vi "Logger.vi"() -> ()   [LabVIEW 2016]
uses:
  tools/CitTemplate/citTemplate.errData.ctl
  Logger.Action.ctl
  Sequence/Sequence.State.ctl
  Sequence/Sequence.Step.Status.ctl
  Sequence/Sequence.UserData.ctl
  Sequence/Sequence.Data.ctl
  tools/EventLog/EventLog.EventSource.ctl
  Sequence/Sequence.MainMode.ctl
  Gui/MainGui.TestOptions.ctl
  Sequence/Sequence.Code.Sets.ctl
  Sequence/Sequence.Prod.StatusData.ctl
  Sequence/Sequence.Test.Unload.Status.ctl
  Sequence/Sequence.Slot.StatusData.ctl
  Sequence/Sequence.Test.Status.ctl
  Sequence/Sequence.Test.BreakReason.ctl
  Sequence/Sequence.UserActions.ctl
  Logger.Variant.Sets.ctl
  Station/Station.Changeover.State.vi
  Sequence/Sequence.Code.SerialFormat.ctl
  Station/Station.Plate.Properties.ctl
  Drivers/V7310/LowLevel/V7310.Job.Sets.ctl
  Sequence/Sequence.PlateType.ctl
  Sequence/Sequence.Counters.ctl
  Sequence/Sequence.Test.BreakSource.ctl
panel:
  out "Folder":string
  out "_loop":i32(ring)=4
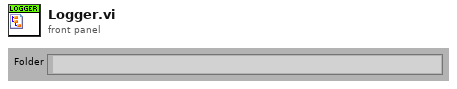
[diagram p1: front panel]
types:
  T1 = typedef "citTemplate.errData.ctl" = cluster{"ts":timestamp, "src":T2, "instance":i32, "action":string, "error":errorcluster, "unconfirmed":bool}
  T2 = typedef "EventLog.EventSource.ctl" = enum16{"All", "Gui", "Ref", "File", "Arch", "Seq", "CPX", "DB", "Laser", "Scan.P", "Scan.O"}
  T3 = typedef "Sequence.Data.ctl" = cluster{"BeginTS":timestamp, "EndTS":timestamp, "State":T4, "Status.Work":T5, "Status.Process":T5, "Status.Home":T5, "Status.Wabco":T5, "Status.Client":T5, "BreakReason":T6, "BreakSource":T7, "DoorLock":bool, "Status.Prod":T8[], "UserAction":T12, "UserData":T13, "Error":errorcluster, "Code":T16, "Rotations":i32, "ProdIdx":i32, "ProdDone":T8[], "PrintedSerials-Wabco":i32[], "PrintedSerials-Client":i32[], "Counters-Wabco":T23, "Counters-Client":T23}
  T4 = typedef "Sequence.State.ctl" = enum16{"Init", "Idle", "Home", "Work", "Run", "Pause"}
  T5 = typedef "Sequence.Step.Status.ctl" = enum16{"-", "Pending", "Running", "Skipped", "Passed", "Failed", "Done", "Error", "Aborted", "Stopped"}
  T6 = typedef "Sequence.Test.BreakReason.ctl" = enum16{"-", "NOK container", "OK container", "Rev empty", "Rev missing", "Rev wrong", "Fork missing", "Fork wrong", "NOK limit", "Unload failure", "Single slot", "Part done", "Err: Prod move work", "Err: Prod move home", "Err: Prod lift work", "Err: Prod lift home", "Err: Prod Arm Work", "Err: Prod Arm NOK", "Err: Prod Arm OK", "Err: Prod NOK suck", "Err: Prod NOK drop", "Err: Prod OK missing", "Err: Prod OK suck", "Err: Prod OK drop"}
  T7 = typedef "Sequence.Test.BreakSource.ctl" = enum16{"-", "A", "B", "A/B"}
  T8 = typedef "Sequence.Test.Status.ctl" = cluster{"Slot":T9, "A":T11, "B":T11}
  T9 = typedef "Sequence.Slot.StatusData.ctl" = cluster{"ID":i32, "Unload":T10, "TS":timestamp, "duration":u32}
  T10 = typedef "Sequence.Test.Unload.Status.ctl" = enum16{"init", "check NOK", "check OK", "wait on NOK", "wait on OK", "wait on Unload", "done"}
  T11 = typedef "Sequence.Prod.StatusData.ctl" = cluster{"status":T5, "pause":T6, "present":bool, "printed":bool, "scanned":bool, "tuned":bool, "removed":bool, "LaserVariables":string[], "Serial":i32, "ScannerReadOut":string[], "path":path, "corners":cluster{"X":i32, "Y":i32}[], "verification":u8}
  T12 = typedef "Sequence.UserActions.ctl" = cluster{"Stop":bool, "Pause":bool, "Next":bool}
  T13 = typedef "Sequence.UserData.ctl" = cluster{"GuiMode":T14, "Test":T15, "ContinueOrder":bool}
  T14 = typedef "Sequence.MainMode.ctl" = enum16{"Process", "Base", "Order", "Manual", "Logs", "Results", "Stats", "DMC Config"}
  T15 = typedef "MainGui.TestOptions.ctl" = cluster{"IgnoreResults":bool, "IgnoreImages":bool, "ServiceMode":bool}
  T16 = typedef "Sequence.Code.Sets.ctl" = cluster{"Ready":bool, "DoubleOrder":bool, "OrderDone":bool, "AllowSingleSlot":bool, "CheckDM":bool, "ThresholdA":u8, "ThresholdB":u8, "Plate":T17, "ImgPath":path, "Variant":T18}
  T17 = typedef "Sequence.PlateType.ctl" = enum16{"Wabco", "Client"}
  T18 = typedef "Logger.Variant.Sets.ctl" = cluster{"State":T19, "ImgPath":path, "WabcoPlate":string, "WabcoProduct":string, "ClientProduct":string, "ClientPlate":string, "TotalQuantity":u16, "OrderQuantity":u16, "Serial":i32, "Wabco":T20, "Client":T20}
  T19 = typedef "Station.Changeover.State.vi" = enum16{"Init", "Scaning", "NOK", "Wait for ack", "Ready"}
  T20 = typedef "Station.Plate.Properties.ctl" = cluster{"LaserJob":string, "AdditionalTxt":string, "FactoryCode":string, "RevID":u8, "ForkID":u8, "FailuresLimit":u16, "GlobalCnt":i32, "Bank":u8, "SerialFormat":T21, "CoordA":T22, "CoordB":T22, "DMCconfig":i32}
  T21 = typedef "Sequence.Code.SerialFormat.ctl" = enum8{"", "6 dig", "7 dig"}
  T22 = typedef "V7310.Job.Sets.ctl" = cluster{"X":dbl, "Y":dbl, "Angle":dbl}
  T23 = typedef "Sequence.Counters.ctl" = cluster{"Expected":u16, "Done":u16, "OK":u16, "NOK":u16, "NOKlimit":u16, "Part":u16, "PartOK":u16}
  T24 = typedef "Logger.Action.ctl" = enum32{"idle", "constructor", "destructor", "--- Logger ---", "Begin", "Add", "End"}
  T25 = typedef "citTemplate.notifierHandle.ctl" = refnum<notifier>
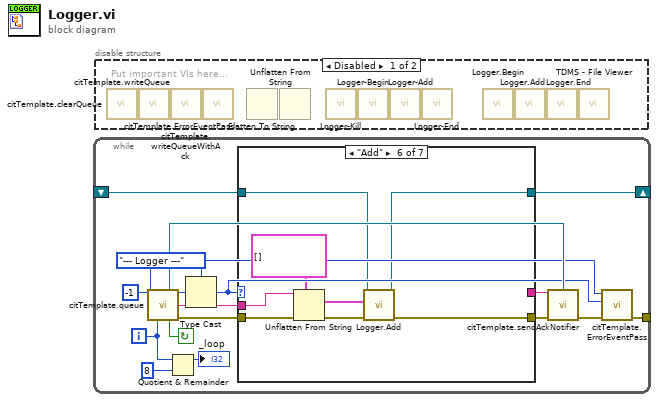
[diagram p0: block diagram]
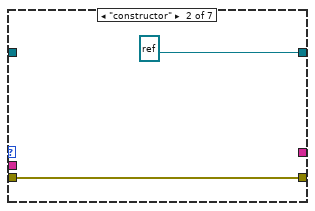
[diagram p4: hidden frame]
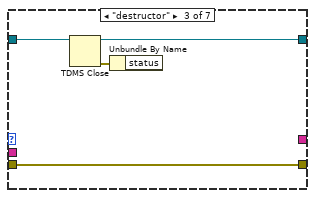
[diagram p5: hidden frame]
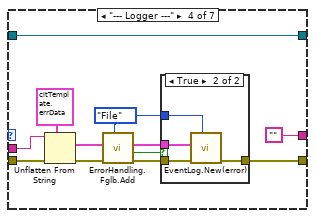
[diagram p6: hidden frame]
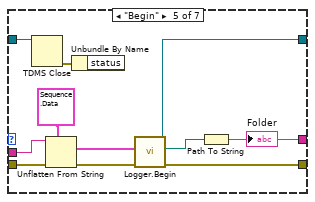
[diagram p8: hidden frame]
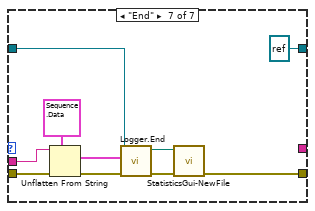
[diagram p9: hidden frame]
diagram:
  n1 = while {
    tunnel: [w4] -> _
    shift-right: [w2] -> _
    shift-left: _ -> [w1]
    i -> [w6]
    stop <- w13 continue-if-true
    w10 = Logger.Action."--- Logger ---" ("Action")
    n2 = call "citTemplate.queue.vi"("ms timeout (250 ms)"=-1, "event enum"=w10, "iteration (-1)"=w6) -> ("notifierHandle out"=w12:T25, "event out"=w16:u32, "(flatten) data out"=w15:string, "continue"=w13:bool, "error out"=w14:errorcluster)  [unwired: 2 in, 6 out]
    n3 = Quotient & Remainder(x=w6, y=8) -> (x-y*floor(x/y)=→"_loop":i32)  [unwired: 1 out]
    n4 = Type Cast(type=w10, x=w16) -> (*(type *) &x=w5:T24)
    n5 = case shown="\"Add\"" w5 {
      tunnel: w15 -> [_ _ _ w33 w49 w57 w67]
      tunnel: w14 -> [w18 w20 w23 w32 w50 w58 w68]
      tunnel: [_ _ _ "" w40 _ _] -> w11
      tunnel: [w18 w20 w23 w25 w47 w55 w60] -> w9
      tunnel: [w17 refnum<k34> refnum ("Refnum out") w22 w24 w42 w53 refnum<k34> refnum ("Refnum out")] -> w2
      tunnel: w1 -> [w17 _ w22 w24 w45 w54 w63]
      frame "idle" {
      }
      frame "constructor" {
      }
      frame "destructor" {
        n6 = TDMS Close(11:w22) -> (0:w21:errorcluster)  [unwired: 1 in, 1 out]
        n7 = Unbundle By Name(w21) -> ()  [unwired: 1 out]
      }
      frame "--- Logger ---" {
        w26 = EventLog.EventSource."File" ("Event source")
        n8 = Unflatten From String(type=T1 {"ts"=timestamp(0 s since 1904-01-01), "src"=enum."All", "instance"=0, "action"="", "error"={"status"=FALSE, "code"=0, "source"=""}, "unconfirmed"=FALSE} ("ErrData"), binary string=w33, error in (no error)=w32) -> (value=w27:T1, error out=w28:errorcluster)  [unwired: 3 out]
        n9 = call "ErrorHandling.Fglb.Add.vi"("Event source"=w26, "error in (no error)"=w28, "Error in"=w27) -> ("error out"=w30:errorcluster, "changed?"=w29:bool)  [unwired: 7 in]
        n10 = case shown="True" w29 {
          tunnel: [w35 w39] -> w25
          tunnel: w27 -> [_ w38]
          tunnel: w30 -> [w35 w37]
          tunnel: w26 -> [_ w36]
          frame False {
          }
          frame True {
            n11 = call "EventLog.New(error).vi"("Source (All)"=w36, "error in"=w37, "ErrData"=w38) -> ("error out"=w39:errorcluster)  [unwired: 8 in]
          }
        }
      }
      frame "Begin" {
        n12 = TDMS Close(11:w45) -> (0:w43:errorcluster)  [unwired: 1 in, 1 out]
        n13 = Unflatten From String(type=T3 {"BeginTS"=timestamp(0 s since 1904-01-01), "EndTS"=timestamp(0 s since 1904-01-01), "State"=enum."Init", "Status.Work"=enum."-", "Status.Process"=enum."-", "Status.Home"=enum."-", "Status.Wabco"=enum."-", "Status.Client"=enum."-", "BreakReason"=enum."-", "BreakSource"=enum."-", "DoorLock"=FALSE, "Status.Prod"=[], "UserAction"={"Stop"=FALSE, "Pause"=FALSE, "Next"=FALSE}, "UserData"={"GuiMode"=enum."Process", "Test"={"IgnoreResults"=FALSE, "IgnoreImages"=FALSE, "ServiceMode"=FALSE}, "ContinueOrder"=FALSE}, "Error"={"status"=FALSE, "code"=0, "source"=""}, "Code"={"Ready"=FALSE, "DoubleOrder"=FALSE, "OrderDone"=FALSE, "AllowSingleSlot"=FALSE, "CheckDM"=FALSE, "ThresholdA"=0, "ThresholdB"=0, "Plate"=enum."Wabco", "ImgPath"=path "", "Variant"={"State"=enum."Init", "ImgPath"=path "", "WabcoPlate"="", "WabcoProduct"="", "ClientProduct"="", "ClientPlate"="", "TotalQuantity"=0, "OrderQuantity"=0, "Serial"=0, "Wabco"={"LaserJob"="", "AdditionalTxt"="", "FactoryCode"="", "RevID"=0, "ForkID"=0, "FailuresLimit"=0, "GlobalCnt"=0, "Bank"=0, "SerialFormat"=enum."", "CoordA"={"X"=0.0, "Y"=0.0, "Angle"=0.0}, "CoordB"={"X"=0.0, "Y"=0.0, "Angle"=0.0}, "DMCconfig"=0}, "Client"={"LaserJob"="", "AdditionalTxt"="", "FactoryCode"="", "RevID"=0, "ForkID"=0, "FailuresLimit"=0, "GlobalCnt"=0, "Bank"=0, "SerialFormat"=enum."", "CoordA"={"X"=0.0, "Y"=0.0, "Angle"=0.0}, "CoordB"={"X"=0.0, "Y"=0.0, "Angle"=0.0}, "DMCconfig"=0}}}, "Rotations"=0, "ProdIdx"=0, "ProdDone"=[], "PrintedSerials-Wabco"=[], "PrintedSerials-Client"=[], "Counters-Wabco"={"Expected"=0, "Done"=0, "OK"=0, "NOK"=0, "NOKlimit"=0, "Part"=0, "PartOK"=0}, "Counters-Client"={"Expected"=0, "Done"=0, "OK"=0, "NOK"=0, "NOKlimit"=0, "Part"=0, "PartOK"=0}} ("Data in"), binary string=w49, error in (no error)=w50) -> (value=w46:T3, error out=w48:errorcluster)  [unwired: 3 out]
        n14 = Unbundle By Name(w43) -> ()  [unwired: 1 out]
        n15 = call "Logger.Begin.vi"("error in"=w48, "Data in"=w46) -> ("error out"=w47:errorcluster, "Folder"=w41:path, "Refnum out"=w42:refnum<k34>)  [unwired: 7 in]
        n16 = Path To String(path=w41) -> (string=w40:string)
        "Folder" <- w40
      }
      frame "Add" {
        n17 = Unflatten From String(type=T8[] [] ("All Slots"), binary string=w57, error in (no error)=w58) -> (value=w52:T8[], error out=w56:errorcluster)  [unwired: 3 out]
        n18 = call "Logger.Add.vi"("error in"=w56, "All Slots"=w52, "Refnum in"=w54) -> ("error out"=w55:errorcluster, "Refnum out"=w53:refnum<k34>)  [unwired: 5 in, 2 out]
      }
      frame "End" {
        n19 = Unflatten From String(type=T3 {"BeginTS"=timestamp(0 s since 1904-01-01), "EndTS"=timestamp(0 s since 1904-01-01), "State"=enum."Init", "Status.Work"=enum."-", "Status.Process"=enum."-", "Status.Home"=enum."-", "Status.Wabco"=enum."-", "Status.Client"=enum."-", "BreakReason"=enum."-", "BreakSource"=enum."-", "DoorLock"=FALSE, "Status.Prod"=[], "UserAction"={"Stop"=FALSE, "Pause"=FALSE, "Next"=FALSE}, "UserData"={"GuiMode"=enum."Process", "Test"={"IgnoreResults"=FALSE, "IgnoreImages"=FALSE, "ServiceMode"=FALSE}, "ContinueOrder"=FALSE}, "Error"={"status"=FALSE, "code"=0, "source"=""}, "Code"={"Ready"=FALSE, "DoubleOrder"=FALSE, "OrderDone"=FALSE, "AllowSingleSlot"=FALSE, "CheckDM"=FALSE, "ThresholdA"=0, "ThresholdB"=0, "Plate"=enum."Wabco", "ImgPath"=path "", "Variant"={"State"=enum."Init", "ImgPath"=path "", "WabcoPlate"="", "WabcoProduct"="", "ClientProduct"="", "ClientPlate"="", "TotalQuantity"=0, "OrderQuantity"=0, "Serial"=0, "Wabco"={"LaserJob"="", "AdditionalTxt"="", "FactoryCode"="", "RevID"=0, "ForkID"=0, "FailuresLimit"=0, "GlobalCnt"=0, "Bank"=0, "SerialFormat"=enum."", "CoordA"={"X"=0.0, "Y"=0.0, "Angle"=0.0}, "CoordB"={"X"=0.0, "Y"=0.0, "Angle"=0.0}, "DMCconfig"=0}, "Client"={"LaserJob"="", "AdditionalTxt"="", "FactoryCode"="", "RevID"=0, "ForkID"=0, "FailuresLimit"=0, "GlobalCnt"=0, "Bank"=0, "SerialFormat"=enum."", "CoordA"={"X"=0.0, "Y"=0.0, "Angle"=0.0}, "CoordB"={"X"=0.0, "Y"=0.0, "Angle"=0.0}, "DMCconfig"=0}}}, "Rotations"=0, "ProdIdx"=0, "ProdDone"=[], "PrintedSerials-Wabco"=[], "PrintedSerials-Client"=[], "Counters-Wabco"={"Expected"=0, "Done"=0, "OK"=0, "NOK"=0, "NOKlimit"=0, "Part"=0, "PartOK"=0}, "Counters-Client"={"Expected"=0, "Done"=0, "OK"=0, "NOK"=0, "NOKlimit"=0, "Part"=0, "PartOK"=0}} ("SeqData"), binary string=w67, error in (no error)=w68) -> (value=w64:T3, error out=w65:errorcluster)  [unwired: 3 out]
        n20 = call "Logger.End.vi"("error in"=w65, "SeqData"=w64, "Refnum in"=w63) -> ("error out"=w61:errorcluster, "File path"=w59:path)  [unwired: 7 in]
        n21 = call "StatisticsGui-NewFile.vi"("error in"=w61, "File"=w59) -> ("error out"=w60:errorcluster)  [unwired: 9 in]
      }
    }
    n22 = call "citTemplate.sendAckNotifier.vi"("notification data"=w11, "notifierHandle in"=w12, "error in"=w9) -> ()  [unwired: 13 out]
    n23 = call "citTemplate.ErrorEventPass.vi"("error in"=w9, "action of error"=w5, "event in"=w10) -> ("error out"=w4:errorcluster)  [unwired: 2 in, 6 out]
  }
  n24 = disable-structure shown="Disabled" {
    frame Disabled {
      # "Put important VIs here..."
      n25 = call "citTemplate.clearQueue.vi"() -> ()  [unwired: 14 in, 2 out]
      n26 = call "citTemplate.writeQueue.vi"() -> ()  [unwired: 15 in, 1 out]
      n27 = call "citTemplate.writeQueueWithAck.vi"() -> ()  [unwired: 13 in, 3 out]
      n28 = call "citTemplate.ErrorEventPass.vi"() -> ()  [unwired: 11 in, 1 out]
      n29 = Flatten To String() -> ()  [unwired: 4 in, 3 out]
      n30 = Unflatten From String() -> ()  [unwired: 5 in, 3 out]
      n31 = call "Logger-Kill.vi"() -> ()  [unwired: 11 in, 1 out]
      n32 = call "Logger-Begin.vi"() -> ()  [unwired: 10 in, 2 out]
      n33 = call "Logger-Add.vi"() -> ()  [unwired: 11 in, 1 out]
      n34 = call "Logger-End.vi"() -> ()  [unwired: 11 in, 1 out]
      n35 = call "Logger.Begin.vi"() -> ()  [unwired: 9 in, 3 out]
      n36 = call "Logger.Add.vi"() -> ()  [unwired: 8 in, 4 out]
      n37 = call "Logger.End.vi"() -> ()  [unwired: 10 in, 2 out]
      n38 = call <vilib>:"TDMS - File Viewer.vi"() -> ()  [unwired: 6 in, 2 out]
    }
    frame Enabled {
    }
  }
